vi "Get Latest Release Version.vi"(8 "error in (no error)":errorcluster, 11 "SelfUpdate in":refnum<class "SelfUpdate.lvclass">) -> (0 "error out":errorcluster, 2 "latest tag":string, 3 "SelfUpdate out":refnum<class "SelfUpdate.lvclass">)   [LabVIEW 2019, in "SelfUpdate.lvclass"]
uses:
  SelfUpdate.lvclass
  SelfUpdate.lvclass/SelfUpdate.ctl
  <vilib>/addons/_JKI.lib/REST Client/classes/REST Client/REST Client.lvclass
  <vilib>/addons/_JKI.lib/REST Client/classes/Response Headers/Response Headers.lvclass
  <vilib>/JKI/JKI SMO/URI Parsing/URI.lvlib
panel:
  out "Value":string
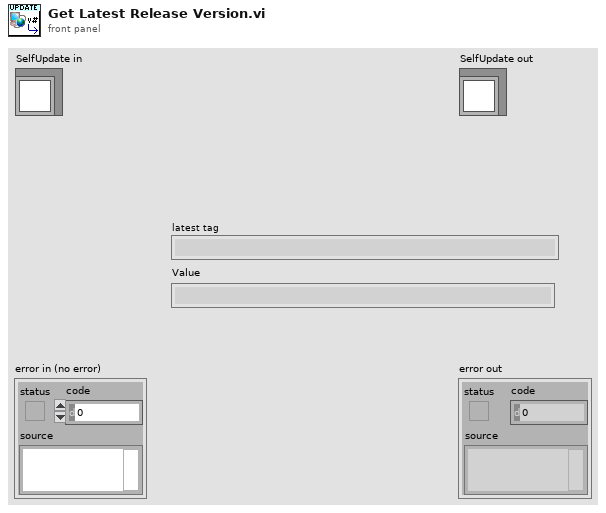
[diagram p1: front panel]
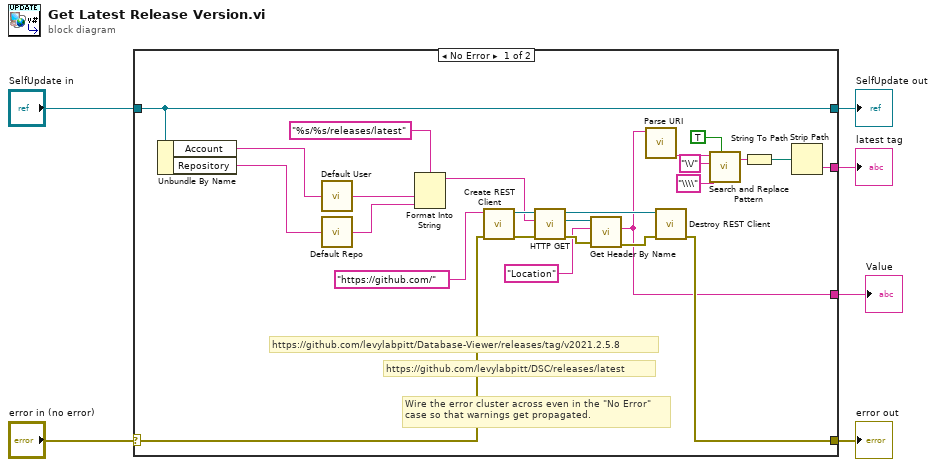
[diagram p0: block diagram]
diagram:
  n1 = case shown="No Error" "error in (no error)" {
    selector: "error in (no error)" -> [w16 w33]
    tunnel: [w15 w33] -> w5
    tunnel: [w31 w32] -> w3
    tunnel: "SelfUpdate in" -> [w31 w32]
    tunnel: [w17 _] -> w2
    tunnel: [w11 _] -> w1
    frame No Error {
      # "https://github.com/levylabpitt/Database-Viewer/releases/tag/v2021.2.5.8"
      # "https://github.com/levylabpitt/DSC/releases/latest"
      # "Wire the error cluster across even in the \"No Error\"\ncase so that warnings get propagated."
      n2 = Unbundle By Name(w31) -> ("Account"=w10:string, "Repository"=w9:string)
      n3 = call "Default User.vi"("Account in"=w10) -> ("Account out"=w7:string)
      n4 = call "Default Repo.vi"("Repo in"=w9) -> ("Repo out"=w8:string)
      n5 = Format Into String(format string="%s/%s/releases/latest", w7, w8) -> (resulting string=w12:string)  [unwired: 2 in, 1 out]
      n6 = call <vilib>:"Create REST Client.vi"("error in (no error)"=w16, "Base URL"="https://github.com/" ("format string")) -> ("error out"=w24:errorcluster, "REST Client out"=w25:refnum<class "REST Client.lvclass">)  [unwired: 8 in]
      n7 = call-dynamic "HTTP GET.vi"("error in (no error)"=w24, "Path"=w12, "REST Client in"=w25) -> ("error out"=w29:errorcluster, "Response Headers"=w30:refnum<class "Response Headers.lvclass">, "REST Client out"=w27:refnum<class "REST Client.lvclass">)  [unwired: 3 in, 3 out]
      n8 = call <vilib>:"Get Header By Name.vi"("error in (no error)"=w29, "Name"="Location", "Response Headers in"=w30) -> ("error out"=w26:errorcluster, "Value"=w11:string)  [unwired: 5 in, 2 out]
      n9 = call <vilib>:"Parse URI.vi"("URI"=w11) -> ("path"=w22:string)  [unwired: 6 in, 4 out]
      n10 = call-dynamic "Destroy REST Client.vi"("error in (no error)"=w26, "REST Client in"=w27) -> ("error out"=w15:errorcluster)  [unwired: 9 in]
      n11 = call <vilib>:"Search and Replace Pattern.vi"("string"=w22, "regular expression (\"\")"="\\/" ("regular expression (\"\")"), "replace string (\"\")"="\\\\" ("replace string (\"\")"), "replace all? (F)"=TRUE) -> ("result string"=w21:string)  [unwired: 1 in, 1 out]
      n12 = String To Path(string=w21) -> (path=w23:path)
      n13 = Strip Path(path=w23) -> (name=w17:string)  [unwired: 1 out]
    }
    frame Error {
    }
  }
  "error out" <- w5
  "SelfUpdate out" <- w3
  "latest tag" <- w2
  "Value" <- w1
